vi "UDPread.vi"(0 "Sender Ip address":string="192.168.0.101") -> (1 "recording Switch":bool, 2 "UDP time of received":string, 3 "UDP read string":string)   [LabVIEW 2017]
panel:
  in  "?":bool
  out "String":string
  in  "Port":u16=61557
  out "error out":errorcluster
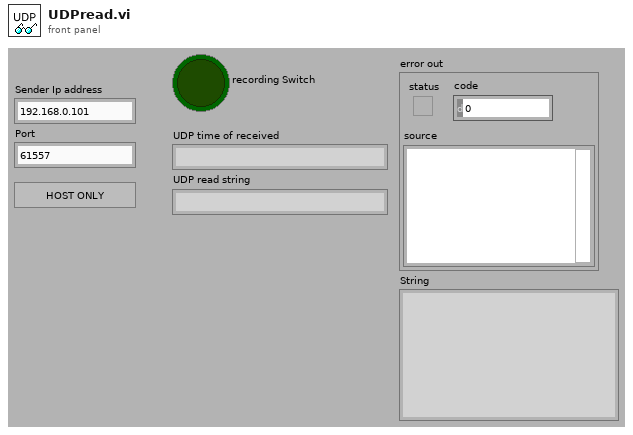
[diagram p1: front panel]
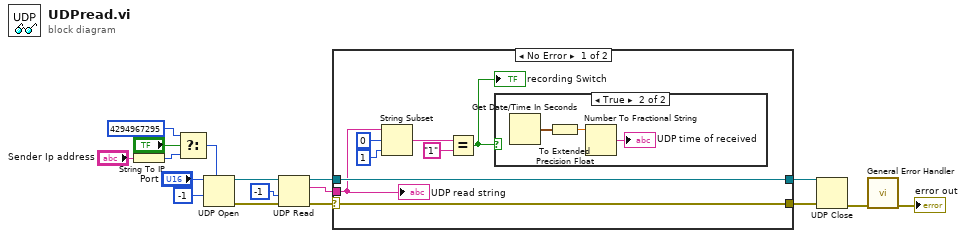
[diagram p0: block diagram]
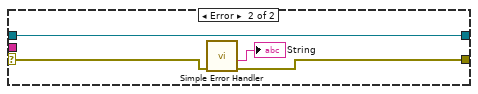
[diagram p3: hidden frame]
diagram:
  n1 = String To IP(1:"Sender Ip address") -> (0:w15:u32)
  n2 = Select(t=u32 4294967295, s="?", f=w15) -> (s? t:f=w13:u32)
  n3 = UDP Open(7:w13, 9:-1, 11:"Port") -> (port=w11:refnum<k16>, 0:w12:errorcluster)  [unwired: 1 in, 2 out]
  n4 = UDP Read(connection ID=w11, timeout ms (25000)=-1, 8:w12) -> (data out=w9:string, error out=w5:errorcluster, 3:w3:refnum<k16>)  [unwired: 3 out]
  n5 = case shown="No Error" w5 {
    selector: w5 -> [w25 w31]
    tunnel: w9 -> [w20 _]
    tunnel: [w25 w30] -> w4
    tunnel: [w24 w29] -> w2
    tunnel: w3 -> [w24 w29]
    frame No Error {
      n6 = String Subset(string=w20, offset (0)=0, length (rest)=1) -> (substring=w23:string)
      n7 = Equal?(x=w23, y="1") -> (x = y?=w18:bool)
      "recording Switch" <- w18
      n8 = case shown="True" w18 {
        frame False {
        }
        frame True {
          n9 = Get Date/Time In Seconds() -> (seconds since 1Jan1904=w26:timestamp)
          n10 = To Extended Precision Float(1:w26) -> (0:w28:ext)
          n11 = Number To Fractional String(number=w28) -> (F-format string=→"UDP time of received":string)  [unwired: 3 out]
        }
      }
      "UDP read string" <- w20
    }
    frame Error {
      n12 = call <vilib>:"Simple Error Handler.vi"("error in (no error)"=w31) -> ("source out"=→"String":string, "error out"=w30:errorcluster)  [unwired: 1 in, 6 out]
    }
  }
  n13 = UDP Close(connection ID=w2, 8:w4) -> (error out=w6:errorcluster)  [unwired: 1 out]
  n14 = call <vilib>:"General Error Handler.vi"("error in (no error)"=w6) -> ("error out"=→"error out":errorcluster)  [unwired: 2 in, 12 out]
